vi "SetTests.vi"(8 "error in (no error)":errorcluster, 10 "Tests":T1[](array[typedef]), 11 "reference in":refnum<class "TestView_Tree_Single.lvclass">) -> (0 "error out":errorcluster, 3 "reference in":refnum<class "TestView_Tree_Single.lvclass">)   [LabVIEW 2022 SP3, in "TestView_Tree_Single.lvlib" / "TestView_Tree_Single.lvclass"]
uses:
  TestView_Tree_Single.lvclass
  Components/MES_Base.lvlibp/Controls/Test.ctl
  TestType.ctl
  <userlib>/_OpenG.lib/string/string.llb/Trim Whitespace (String Array)__ogtk.vi
  <userlib>/_OpenG.lib/string/string.llb/Trim Whitespace (String)__ogtk.vi
  Components/MES_Base.lvlibp/MES_Base.lvclass
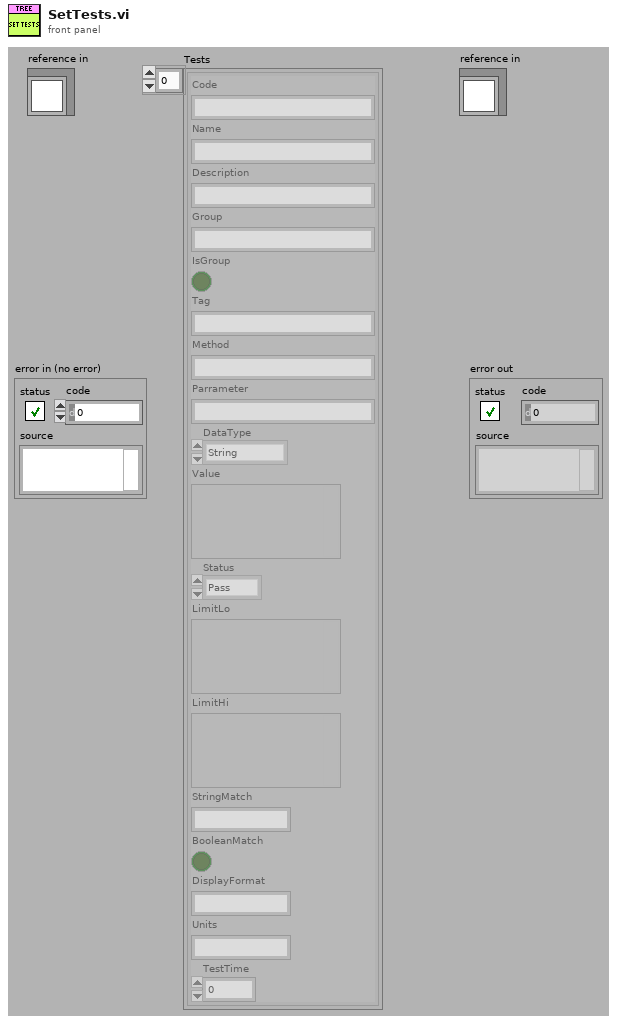
[diagram p1: front panel]
types:
  T1 = typedef "MES_Base.lvlibp/MES_Base.lvclass/Test.ctl" = cluster{"Code":string, "Name":string, "Description":string, "Group":string, "IsGroup":bool, "Tag":string, "Method":string, "Parrameter":string, "DataType":enum16{"NA", "String", "Boolean", "Int", "Dbl"}, "Value":variant, "Status":enum16{"Pending", "Pass", "Fail"}, "LimitLo":variant, "LimitHi":variant, "StringMatch":string, "BooleanMatch":bool, "DisplayFormat":string, "Units":string, "TestTime":dbl}
  T2 = typedef "TestView_Tree_Single.lvlib/TestView_Tree_Single.lvclass/TestType.ctl" = enum16{"null", "action", "action_active", "action_done", "group", "group_active", "group_fail", "group_pass", "test", "test_active", "test_fail", "test_pass", "warning"}
  T3 = typedef "TestView_Tree_Single.lvlib/TestView_Tree_Single.lvclass/ObjectAttributes.ctl" = cluster{"Front Panel":refnum<vi>, "Last_Item":string, "Config":T4, "Title":string, "User":string, "TreeRef":refnum<vi>, "Active DUT":i32, "Status":T5, "SN":string, "Spec":string}
  T4 = typedef "TestView_Tree_Single.lvlib/TestView_Tree_Single.lvclass/Config.ctl" = cluster{"default":string}
  T5 = typedef "TestView_Base.lvlibp/TestView_Base.lvclass/ViewStatus.ctl" = enum16{"Testing", "Ready", "Logout", "Login", "PASS", "FAIL", "FAULT", "ABORTED"}
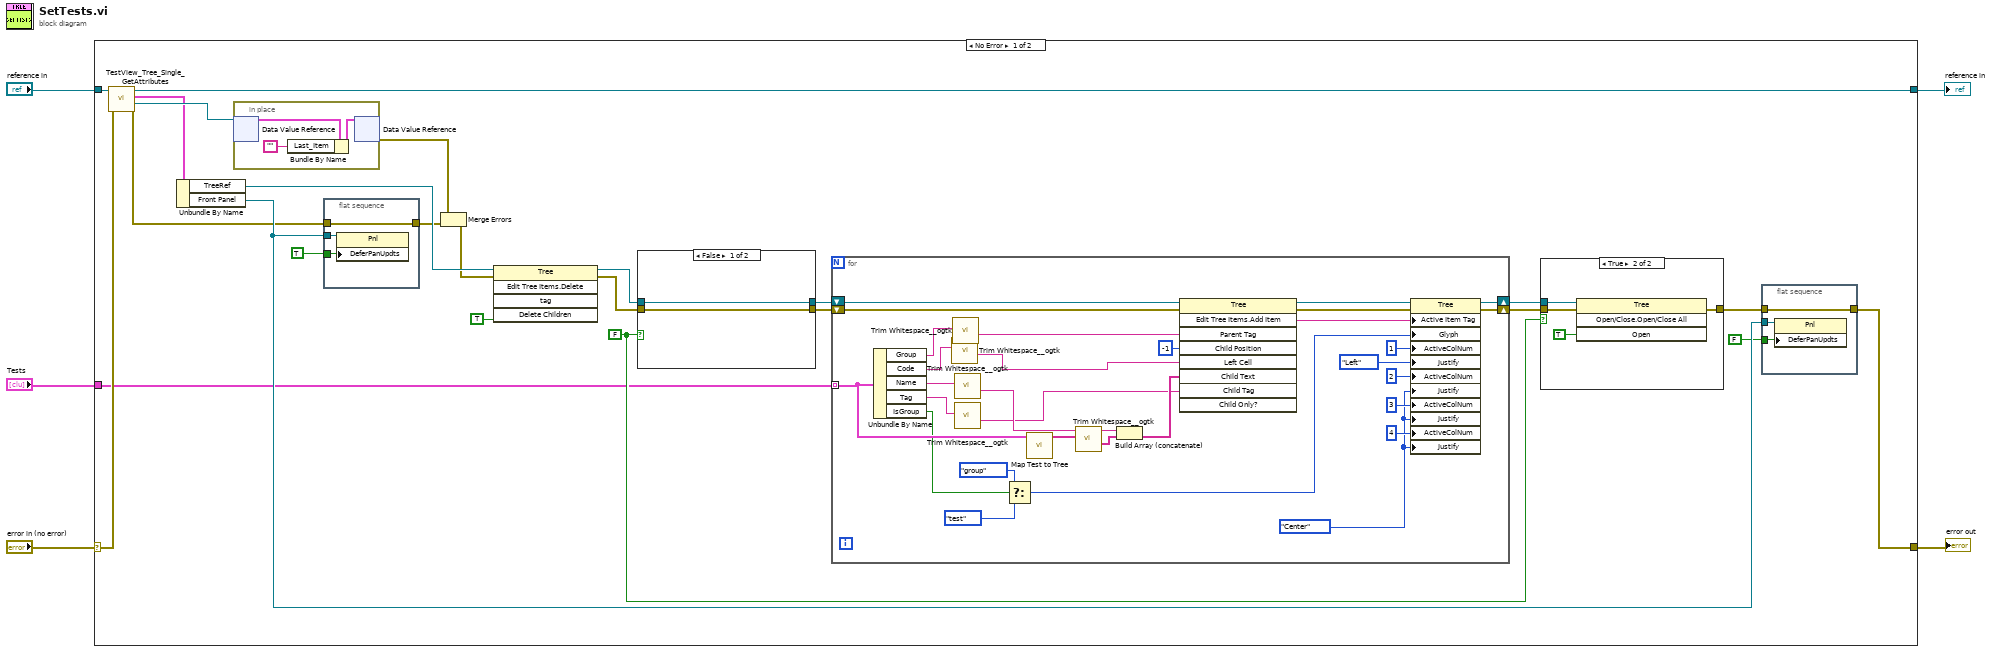
[diagram p0: block diagram]
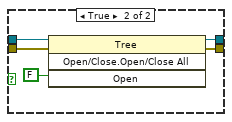
[diagram p3: hidden frame]
diagram:
  n1 = case shown="No Error" "error in (no error)" {
    selector: "error in (no error)" -> [w27 w82]
    tunnel: [w21 w82] -> w4
    tunnel: [w28 w81] -> w2
    tunnel: "reference in" -> [w29 w81]
    tunnel: "Tests" -> [w6 _]
    frame No Error {
      w7 = FALSE
      n2 = call "TestView_Tree_Single_GetAttributes.vi"("error in (no error)"=w27, "reference in"=w29) -> ("error out"=w22:errorcluster, "DataRef"=w26:refnum<data-value>, "Data"=w25:T3, "reference out"=w28:refnum<class "TestView_Tree_Single.lvclass">)  [unwired: 6 in]
      n3 = Unbundle By Name(w25) -> ("TreeRef"=w24:refnum<vi>, "Front Panel"=w23:refnum<vi>)
      n4 = in-place {
        n5 = in-place-dvr #1(w26) -> (w50:T3)  [unwired: 1 out]
        n6 = Bundle By Name(cluster=w50, "Last_Item"="") -> (w49:T3)
        n7 = in-place-dvr #1(w49) -> (w8:errorcluster)  [unwired: 1 out]
      }
      n8 = flat-sequence {
        tunnel: w23 -> [w47]
        tunnel: TRUE ("Defer Panel Updates") -> [w46]
        tunnel: w22 -> [w45]
        tunnel: [w45] -> w9
        frame #0 {
          n9 = property class="Pnl"(reference=w47, "DeferPanUpdts"=w46) -> ()  [unwired: 1 in, 2 out]
        }
      }
      n10 = Merge Errors(w8, w9) -> (w10:errorcluster)
      n11 = invoke class="Tree" method="Edit Tree Items.Delete"(reference=w24, error in=w10, "Delete Children"=TRUE ("Delete Children?")) -> (reference out=w19:refnum<vi>, error out=w18:errorcluster)  [unwired: 2 in, 3 out]
      n12 = case shown="False" w7 {
        tunnel: w19 -> [w35 w41]
        tunnel: w18 -> [w36 w40]
        tunnel: [w36 w39] -> w17
        tunnel: [w35 w38] -> w13
        frame False {
        }
        frame True {
          n13 = invoke class="Tree" method="Open/Close.Open/Close All"(reference=w41, error in=w40, "Open"=FALSE ("Open?")) -> (reference out=w38:refnum<vi>, error out=w39:errorcluster)  [unwired: 1 in, 2 out]
        }
      }
      n14 = for {
        tunnel: w6 -> [w72] mode=indexing
        shift-right: [w76] -> w12
        shift-left: w17 -> [w80]
        shift-right: [w75] -> w11
        shift-left: w13 -> [w79]
        w55 = enum16{"Left", "Center", "Right"}."Center" ("Active Cell:Cell Justification")
        n15 = Unbundle By Name(w72) -> ("Group"=w67:string, "Code"=w65:string, "Name"=w63:string, "Tag"=w61:string, "IsGroup"=w54:bool)
        n16 = call-poly <userlib>:"Trim Whitespace__ogtk.vi"("String in"=w65) -> ("String out"=w64:string)  [unwired: 6 in]
        n17 = call-poly <userlib>:"Trim Whitespace__ogtk.vi"("String in"=w67) -> ("String out"=w66:string)  [unwired: 6 in]
        n18 = call-poly <userlib>:"Trim Whitespace__ogtk.vi"("String in"=w63) -> ("String out"=w62:string)  [unwired: 6 in]
        n19 = call-poly <userlib>:"Trim Whitespace__ogtk.vi"("String in"=w61) -> ("String out"=w60:string)  [unwired: 6 in]
        n20 = Select(t=TestType."group" ("glyph"), s=w54, f=TestType."test" ("glyph")) -> (s? t:f=w51:T2)
        n21 = call "Map Test to Tree.vi"("Test"=w72) -> ("Text"=w59:string[])  [unwired: 7 in, 3 out]
        n22 = call-poly <userlib>:"Trim Whitespace__ogtk.vi"("String in"=w59) -> ("String out"=w58:string[])  [unwired: 6 in]
        n23 = Build Array (concatenate)(w62, w58) -> (w68:string[])
        n24 = invoke class="Tree" method="Edit Tree Items.Add Item"(reference=w79, error in=w80, "Parent Tag"=w66, "Child Position"=-1, "Left Cell"=w64, "Child Text"=w68, "Child Tag"=w60) -> (reference out=w78:refnum<vi>, error out=w77:errorcluster, "Edit Tree Items:Add Item"=w74:string)  [unwired: 2 in, 6 out]
        n25 = property class="Tree"(reference=w78, error in=w77, "Active Item Tag"=w74, "Glyph"=w51, "ActiveColNum"=1 ("Active Cell:Active Column Number"), "Justify"=enum16{"Left", "Center", "Right"}."Left" ("Active Cell:Cell Justification"), "ActiveColNum"=2 ("Active Cell:Active Column Number"), "Justify"=w55, "ActiveColNum"=3 ("Active Cell:Active Column Number"), "Justify"=w55, "ActiveColNum"=4 ("Active Cell:Active Column Number"), "Justify"=w55) -> (reference out=w75:refnum<vi>, error out=w76:errorcluster)
      }
      n26 = case shown="True" w7 {
        tunnel: [w30 w34] -> w14
        tunnel: w12 -> [w30 w33]
        tunnel: w11 -> [_ w32]
        frame False {
        }
        frame True {
          n27 = invoke class="Tree" method="Open/Close.Open/Close All"(reference=w32, error in=w33, "Open"=TRUE ("Open?")) -> (error out=w34:errorcluster)  [unwired: 1 in, 3 out]
        }
      }
      n28 = flat-sequence {
        tunnel: w23 -> [w44]
        tunnel: FALSE ("Defer Panel Updates") -> [w43]
        tunnel: w14 -> [w42]
        tunnel: [w42] -> w21
        frame #0 {
          n29 = property class="Pnl"(reference=w44, "DeferPanUpdts"=w43) -> ()  [unwired: 1 in, 2 out]
        }
      }
    }
    frame Error {
    }
  }
  "error out" <- w4
  "reference in" <- w2
